vi "MeasLeakRate08.vi"() -> ()   [LabVIEW 2011]
panel:
  out "XY Graph":cluster{"Value":dbl[], "Value":dbl[]}(graph)
  in  "Control Valve local":bool
  in  "Exhaust Local":bool
  in  "Exhaust Close":bool
  in  "Exhaust Open":bool
  in  "Control Close":bool
  in  "Control Open":bool
  in  "reset":bool
  in  "# points to watch":i32=60
  out "leak rate (Torr/min)":string
  out "S20":dbl
  out "S11":dbl
  out "S10":dbl
  out "S01":dbl
  out "S00":dbl
  out "A11":dbl[](array[numeric])
  out "P":dbl
  in  "first":bool=TRUE
  out "A20":dbl[](array[numeric])
  out "A10":dbl[](array[numeric])
  out "A01":dbl[](array[numeric])
  out "A00":dbl[](array[numeric])
  in  "interval (s)":dbl=0.5
  in  "stop":bool
  out "P(Torr)":string
  # "Pressure control valve:"
  # "Exahaust valve:"
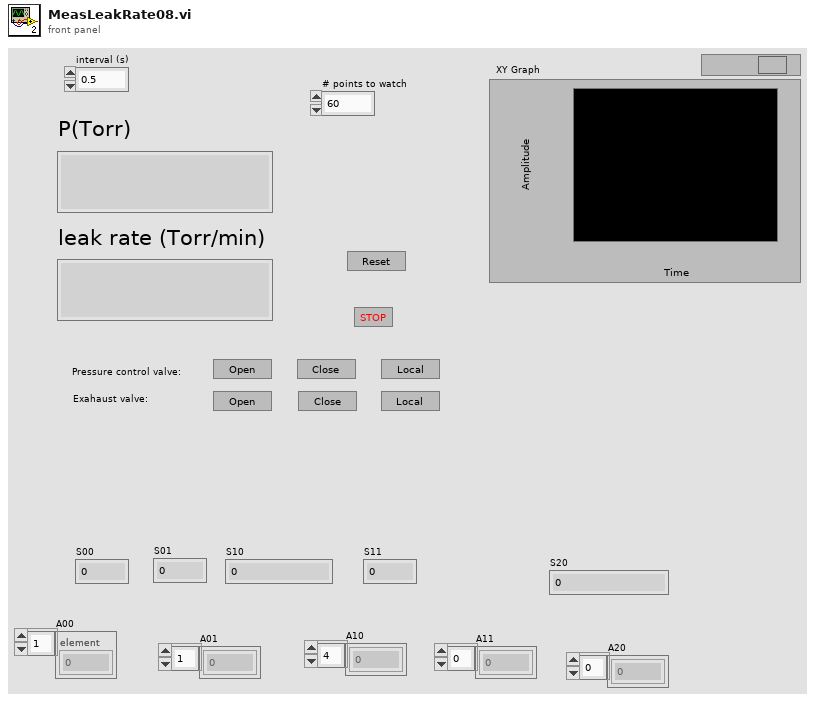
[diagram p1: front panel]
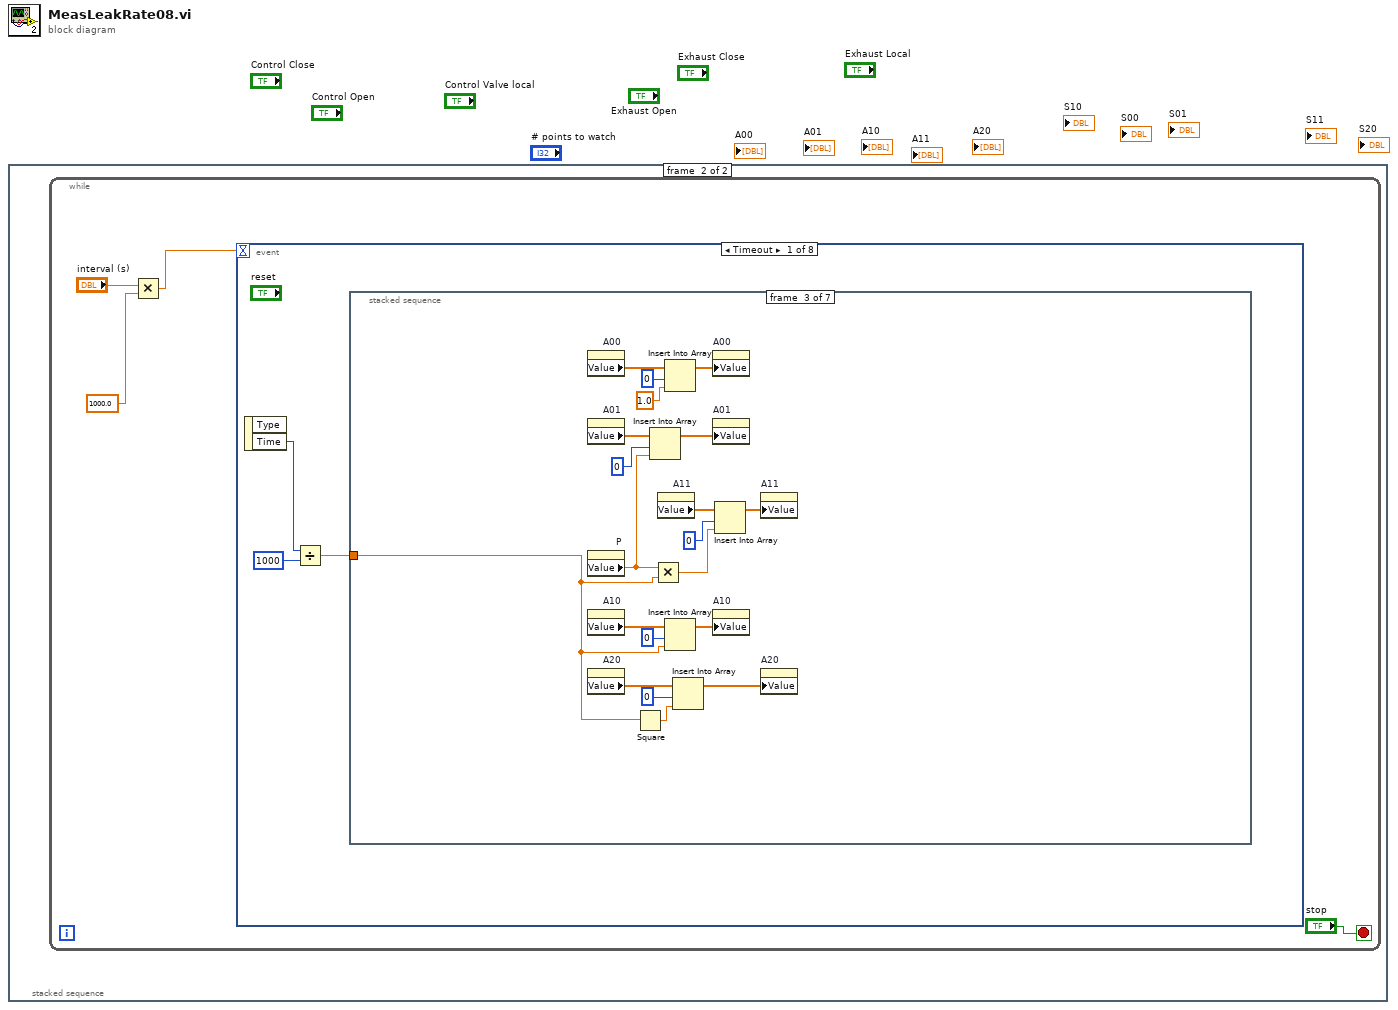
[diagram p0: block diagram]
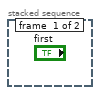
[diagram p2: hidden frame]
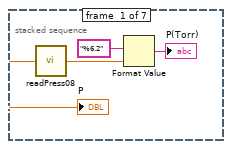
[diagram p3: hidden frame]
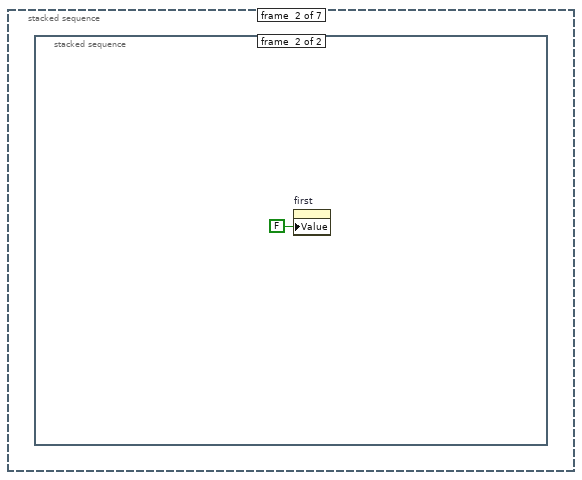
[diagram p4: hidden frame]
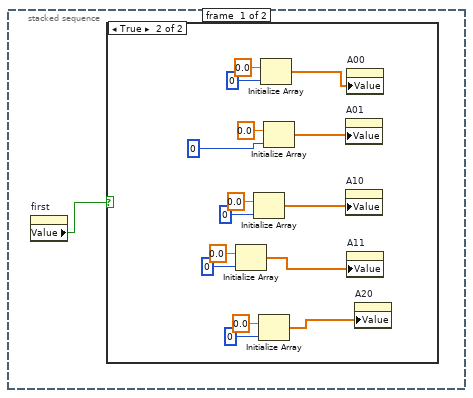
[diagram p5: hidden frame]
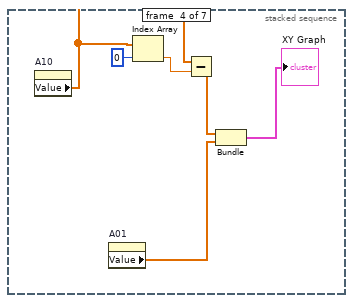
[diagram p7: hidden frame]
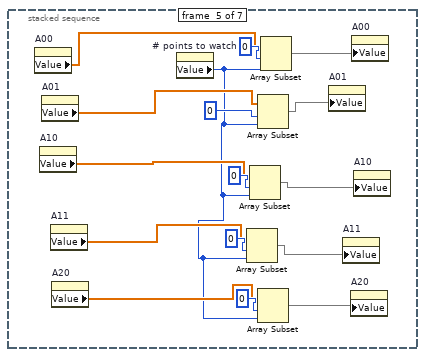
[diagram p8: hidden frame]
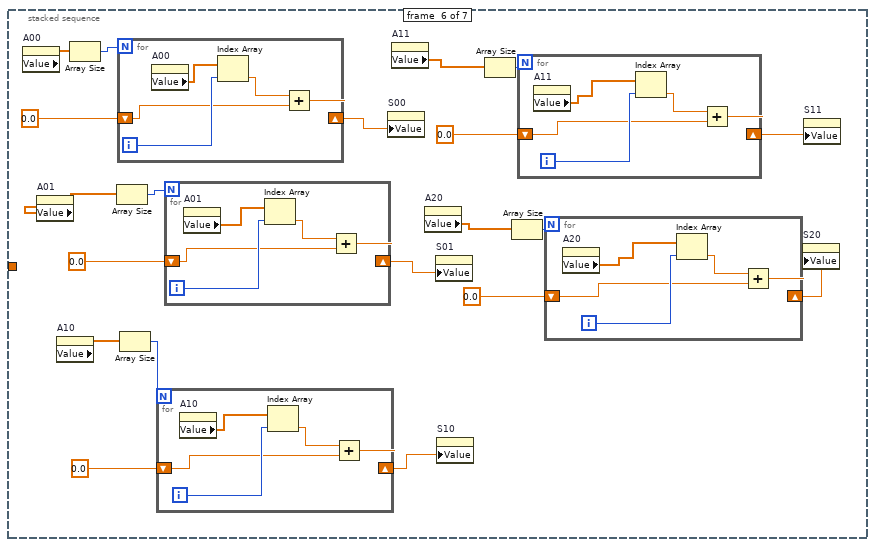
[diagram p9: hidden frame]
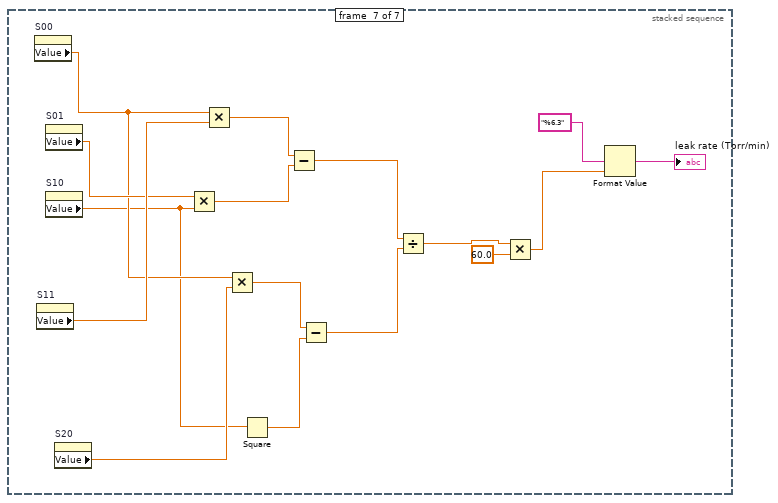
[diagram p10: hidden frame]
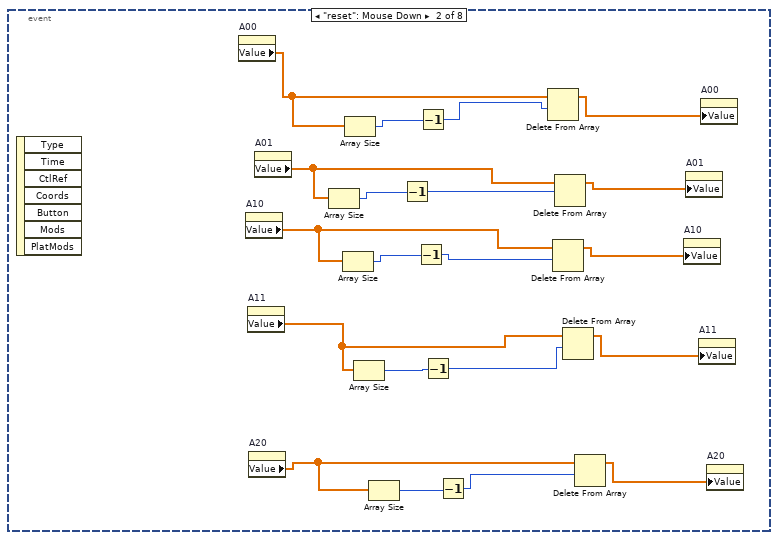
[diagram p11: hidden frame]
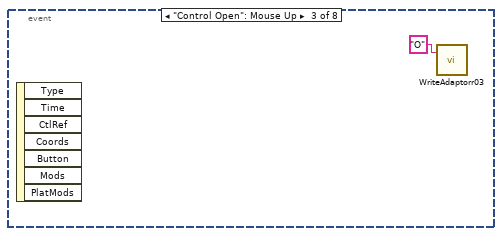
[diagram p12: hidden frame]
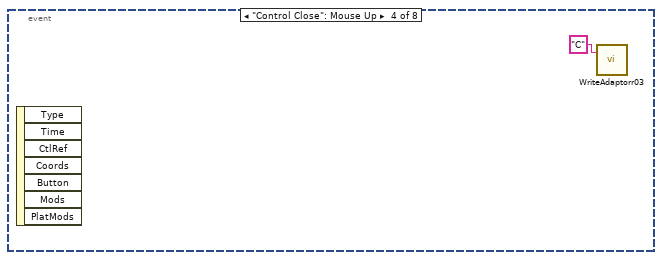
[diagram p13: hidden frame]
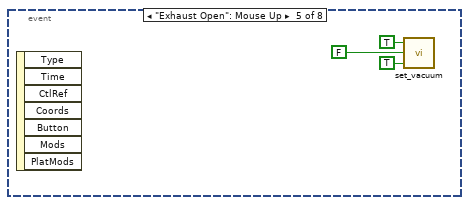
[diagram p14: hidden frame]
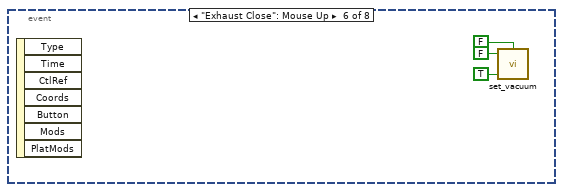
[diagram p15: hidden frame]
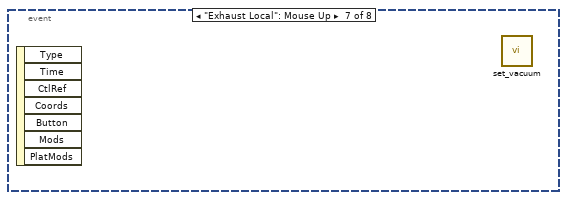
[diagram p16: hidden frame]
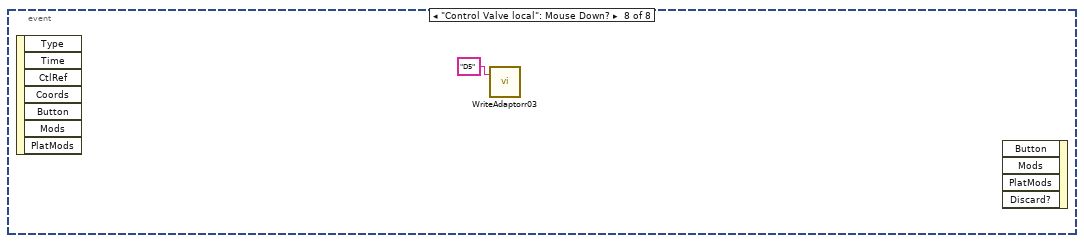
[diagram p17: hidden frame]
diagram:
  n1 = stacked-sequence {
    frame #0 {
    }
    frame #1 {
      n2 = while {
        stop <- "stop" stop-if-true
        n3 = Multiply(x="interval (s)", y=1000.0) -> (x*y=w2:dbl)
        n4 = event shown="[0] Timeout" {
          selector: _ -> [_ _ _ _ _ _ _ _]
          dyn-events: _ -> [_ _ _ _ _ _ _ _]
          timeout: w2 -> [_ _ _ _ _ _ _ _]
          event Timeout {
            n5 = event-data() -> ("Time"=w7:u32)  [unwired: 1 in, 1 out]
            n6 = Divide(x=w7, y=u32 1000) -> (x/y=w5:dbl)
            n7 = stacked-sequence {
              tunnel: w5 -> [_ _ w37 _ _ _ _]
              frame #0 {
                n8 = call "readPress08.vi"() -> ("P"=w9:dbl)
                "P" <- w9
                n9 = Format Value(format string="%6.2", value (0)=w9) -> (output string=→"P(Torr)":string)  [unwired: 1 in]
              }
              frame #1 {
                n10 = stacked-sequence {
                  frame #0 {
                    n11 = property on="first" class="Bool (strict)"() -> ("Value"=w11:bool)  [unwired: 2 in, 2 out]
                    n12 = case shown="True" w11 {
                      frame False {
                      }
                      frame True {
                        n13 = Initialize Array(0.0 ("element"), 0 ("dimension size")) -> (w14:dbl[])
                        n14 = Initialize Array(0.0 ("element"), 0 ("dimension size")) -> (w15:dbl[])
                        n15 = Initialize Array(0.0 ("element"), 0 ("dimension size")) -> (w13:dbl[])
                        n16 = Initialize Array(0.0 ("element"), 0 ("dimension size")) -> (w12:dbl[])
                        n17 = Initialize Array(0.0 ("element"), 0 ("dimension size")) -> (w16:dbl[])
                        n18 = property on="A01" class="Arr (strict)"("Value"=w16) -> ()  [unwired: 2 in, 2 out]
                        n19 = property on="A10" class="Arr (strict)"("Value"=w15) -> ()  [unwired: 2 in, 2 out]
                        n20 = property on="A00" class="Arr (strict)"("Value"=w12) -> ()  [unwired: 2 in, 2 out]
                        n21 = property on="A11" class="Arr (strict)"("Value"=w14) -> ()  [unwired: 2 in, 2 out]
                        n22 = property on="A20" class="Arr (strict)"("Value"=w13) -> ()  [unwired: 2 in, 2 out]
                      }
                    }
                  }
                  frame #1 {
                    n23 = property on="first" class="Bool (strict)"("Value"=FALSE ("first")) -> ()  [unwired: 2 in, 2 out]
                  }
                }
              }
              frame #2 {
                n24 = property on="A00" class="Arr (strict)"() -> ("Value"=w45:dbl[])  [unwired: 2 in, 2 out]
                n25 = property on="A01" class="Arr (strict)"() -> ("Value"=w43:dbl[])  [unwired: 2 in, 2 out]
                n26 = property on="P" class="DigNum (strict)"() -> ("Value"=w36:dbl)  [unwired: 2 in, 2 out]
                n27 = property on="A10" class="Arr (strict)"() -> ("Value"=w42:dbl[])  [unwired: 2 in, 2 out]
                n28 = property on="A20" class="Arr (strict)"() -> ("Value"=w40:dbl[])  [unwired: 2 in, 2 out]
                n29 = Square(x=w37) -> (x^2=w38:dbl)
                n30 = Insert Into Array(array=w43, index=0, new element=w36) -> (w28:dbl[])
                n31 = Multiply(x=w36, y=w37) -> (x*y=w34:dbl)
                n32 = property on="A11" class="Arr (strict)"() -> ("Value"=w35:dbl[])  [unwired: 2 in, 2 out]
                n33 = Insert Into Array(array=w45, index=0, new element=1.0 ("new element/subarray")) -> (w32:dbl[])
                n34 = Insert Into Array(array=w42, index=0, new element=w37) -> (w30:dbl[])
                n35 = Insert Into Array(array=w40, index=0, new element=w38) -> (w31:dbl[])
                n36 = property on="A00" class="Arr (strict)"("Value"=w32) -> ()  [unwired: 2 in, 2 out]
                n37 = property on="A01" class="Arr (strict)"("Value"=w28) -> ()  [unwired: 2 in, 2 out]
                n38 = property on="A10" class="Arr (strict)"("Value"=w30) -> ()  [unwired: 2 in, 2 out]
                n39 = Insert Into Array(array=w35, index=0, new element=w34) -> (w29:dbl[])
                n40 = property on="A11" class="Arr (strict)"("Value"=w29) -> ()  [unwired: 2 in, 2 out]
                n41 = property on="A20" class="Arr (strict)"("Value"=w31) -> ()  [unwired: 2 in, 2 out]
              }
              frame #3 {
                n42 = property on="A10" class="Arr (strict)"() -> ("Value"=w49:dbl[])  [unwired: 2 in, 2 out]
                n43 = property on="A01" class="Arr (strict)"() -> ("Value"=w52:dbl[])  [unwired: 2 in, 2 out]
                n44 = Index Array(array=w49, index=0) -> (element=w50:dbl)
                n45 = Subtract(x=w49, y=w50) -> (x-y=w48:dbl[])
                n46 = Bundle(w48, "Value"=w52) -> (→"XY Graph":cluster{dbl[], "Value":dbl[]})  [unwired: 1 in]
              }
              frame #4 {
                n47 = property on="A00" class="Arr (strict)"() -> ("Value"=w66:dbl[])  [unwired: 2 in, 2 out]
                n48 = property on="A10" class="Arr (strict)"() -> ("Value"=w60:dbl[])  [unwired: 2 in, 2 out]
                n49 = property on="A01" class="Arr (strict)"() -> ("Value"=w61:dbl[])  [unwired: 2 in, 2 out]
                n50 = property on="A11" class="Arr (strict)"() -> ("Value"=w59:dbl[])  [unwired: 2 in, 2 out]
                n51 = property on="A20" class="Arr (strict)"() -> ("Value"=w68:dbl[])  [unwired: 2 in, 2 out]
                n52 = property on="# points to watch" class="DigNum (strict)"() -> ("Value"=w54:i32)  [unwired: 2 in, 2 out]
                n53 = Array Subset(array=w59, index=0, length=w54) -> (w56:dbl[])
                n54 = Array Subset(array=w60, index=0, length=w54) -> (w57:dbl[])
                n55 = Array Subset(array=w61, index=0, length=w54) -> (w58:dbl[])
                n56 = Array Subset(array=w68, index=0, length=w54) -> (w55:dbl[])
                n57 = Array Subset(array=w66, index=0, length=w54) -> (w65:dbl[])
                n58 = property on="A01" class="Arr (strict)"("Value"=w58) -> ()  [unwired: 2 in, 2 out]
                n59 = property on="A11" class="Arr (strict)"("Value"=w56) -> ()  [unwired: 2 in, 2 out]
                n60 = property on="A20" class="Arr (strict)"("Value"=w55) -> ()  [unwired: 2 in, 2 out]
                n61 = property on="A00" class="Arr (strict)"("Value"=w65) -> ()  [unwired: 2 in, 2 out]
                n62 = property on="A10" class="Arr (strict)"("Value"=w57) -> ()  [unwired: 2 in, 2 out]
              }
              frame #5 {
                n63 = property on="A00" class="Arr (strict)"() -> ("Value"=w88:dbl[])  [unwired: 2 in, 2 out]
                n64 = property on="A01" class="Arr (strict)"() -> ("Value"=w84:dbl[])  [unwired: 2 in, 2 out]
                n65 = property on="A10" class="Arr (strict)"() -> ("Value"=w81:dbl[])  [unwired: 2 in, 2 out]
                n66 = Array Size(array=w88) -> (size(s)=w89:i32)
                n67 = Array Size(array=w84) -> (size(s)=w86:i32)
                n68 = for {
                  N: w89 -> [_]
                  shift-right: [w110] -> w74
                  shift-left: 0.0 -> [w111]
                  i -> [w113]
                  n69 = property on="A00" class="Arr (strict)"() -> ("Value"=w114:dbl[])  [unwired: 2 in, 2 out]
                  n70 = Index Array(array=w114, index=w113) -> (element=w112:dbl)
                  n71 = Add(x=w112, y=w111) -> (x+y=w110:dbl)
                }
                n72 = Array Size(array=w81) -> (size(s)=w83:i32)
                n73 = for {
                  N: w83 -> [_]
                  shift-right: [w101] -> w73
                  shift-left: 0.0 -> [w102]
                  i -> [w104]
                  n74 = property on="A10" class="Arr (strict)"() -> ("Value"=w100:dbl[])  [unwired: 2 in, 2 out]
                  n75 = Index Array(array=w100, index=w104) -> (element=w103:dbl)
                  n76 = Add(x=w103, y=w102) -> (x+y=w101:dbl)
                }
                n77 = for {
                  N: w86 -> [_]
                  shift-right: [w106] -> w72
                  shift-left: 0.0 -> [w107]
                  i -> [w109]
                  n78 = property on="A01" class="Arr (strict)"() -> ("Value"=w105:dbl[])  [unwired: 2 in, 2 out]
                  n79 = Index Array(array=w105, index=w109) -> (element=w108:dbl)
                  n80 = Add(x=w108, y=w107) -> (x+y=w106:dbl)
                }
                n81 = property on="S00" class="DigNum (strict)"("Value"=w74) -> ()  [unwired: 2 in, 2 out]
                n82 = property on="A11" class="Arr (strict)"() -> ("Value"=w78:dbl[])  [unwired: 2 in, 2 out]
                n83 = property on="A20" class="Arr (strict)"() -> ("Value"=w75:dbl[])  [unwired: 2 in, 2 out]
                n84 = property on="S01" class="DigNum (strict)"("Value"=w72) -> ()  [unwired: 2 in, 2 out]
                n85 = property on="S10" class="DigNum (strict)"("Value"=w73) -> ()  [unwired: 2 in, 2 out]
                n86 = Array Size(array=w78) -> (size(s)=w80:i32)
                n87 = Array Size(array=w75) -> (size(s)=w77:i32)
                n88 = for {
                  N: w80 -> [_]
                  shift-right: [w96] -> w71
                  shift-left: 0.0 -> [w97]
                  i -> [w99]
                  n89 = property on="A11" class="Arr (strict)"() -> ("Value"=w95:dbl[])  [unwired: 2 in, 2 out]
                  n90 = Index Array(array=w95, index=w99) -> (element=w98:dbl)
                  n91 = Add(x=w98, y=w97) -> (x+y=w96:dbl)
                }
                n92 = for {
                  N: w77 -> [_]
                  shift-right: [w91] -> w70
                  shift-left: 0.0 -> [w92]
                  i -> [w94]
                  n93 = property on="A20" class="Arr (strict)"() -> ("Value"=w90:dbl[])  [unwired: 2 in, 2 out]
                  n94 = Index Array(array=w90, index=w94) -> (element=w93:dbl)
                  n95 = Add(x=w93, y=w92) -> (x+y=w91:dbl)
                }
                n96 = property on="S20" class="DigNum (strict)"("Value"=w70) -> ()  [unwired: 2 in, 2 out]
                n97 = property on="S11" class="DigNum (strict)"("Value"=w71) -> ()  [unwired: 2 in, 2 out]
              }
              frame #6 {
                n98 = property on="S00" class="DigNum (strict)"() -> ("Value"=w126:dbl)  [unwired: 2 in, 2 out]
                n99 = property on="S11" class="DigNum (strict)"() -> ("Value"=w130:dbl)  [unwired: 2 in, 2 out]
                n100 = property on="S01" class="DigNum (strict)"() -> ("Value"=w129:dbl)  [unwired: 2 in, 2 out]
                n101 = property on="S10" class="DigNum (strict)"() -> ("Value"=w124:dbl)  [unwired: 2 in, 2 out]
                n102 = property on="S20" class="DigNum (strict)"() -> ("Value"=w125:dbl)  [unwired: 2 in, 2 out]
                n103 = Multiply(x=w129, y=w124) -> (x*y=w127:dbl)
                n104 = Multiply(x=w126, y=w130) -> (x*y=w128:dbl)
                n105 = Multiply(x=w126, y=w125) -> (x*y=w123:dbl)
                n106 = Square(x=w124) -> (x^2=w122:dbl)
                n107 = Subtract(x=w128, y=w127) -> (x-y=w121:dbl)
                n108 = Subtract(x=w123, y=w122) -> (x-y=w120:dbl)
                n109 = Divide(x=w121, y=w120) -> (x/y=w119:dbl)
                n110 = Multiply(x=w119, y=60.0) -> (x*y=w115:dbl)
                n111 = Format Value(format string="%6.3", value (0)=w115) -> (output string=→"leak rate (Torr/min)":string)  [unwired: 1 in]
              }
            }
          }
          event "reset": Mouse Down {
            n112 = event-data() -> ()  [unwired: 1 in, 7 out]
            n113 = property on="A00" class="Arr (strict)"() -> ("Value"=w150:dbl[])  [unwired: 2 in, 2 out]
            n114 = property on="A10" class="Arr (strict)"() -> ("Value"=w143:dbl[])  [unwired: 2 in, 2 out]
            n115 = property on="A11" class="Arr (strict)"() -> ("Value"=w140:dbl[])  [unwired: 2 in, 2 out]
            n116 = property on="A20" class="Arr (strict)"() -> ("Value"=w137:dbl[])  [unwired: 2 in, 2 out]
            n117 = property on="A01" class="Arr (strict)"() -> ("Value"=w146:dbl[])  [unwired: 2 in, 2 out]
            n118 = Array Size(array=w146) -> (size(s)=w145:i32)
            n119 = Array Size(array=w143) -> (size(s)=w142:i32)
            n120 = Array Size(array=w150) -> (size(s)=w148:i32)
            n121 = Array Size(array=w140) -> (size(s)=w139:i32)
            n122 = Array Size(array=w137) -> (size(s)=w136:i32)
            n123 = Decrement(x=w145) -> (x-1=w144:i32)
            n124 = Decrement(x=w142) -> (x-1=w141:i32)
            n125 = Decrement(x=w148) -> (x-1=w147:i32)
            n126 = Decrement(x=w139) -> (x-1=w138:i32)
            n127 = Decrement(x=w136) -> (x-1=w135:i32)
            n128 = Delete From Array(array=w150, length=w147) -> (array with subset deleted=w149:dbl[])  [unwired: 1 in, 1 out]
            n129 = Delete From Array(array=w143, length=w141) -> (array with subset deleted=w133:dbl[])  [unwired: 1 in, 1 out]
            n130 = Delete From Array(array=w146, length=w144) -> (array with subset deleted=w134:dbl[])  [unwired: 1 in, 1 out]
            n131 = Delete From Array(array=w140, length=w138) -> (array with subset deleted=w132:dbl[])  [unwired: 1 in, 1 out]
            n132 = Delete From Array(array=w137, length=w135) -> (array with subset deleted=w131:dbl[])  [unwired: 1 in, 1 out]
            n133 = property on="A10" class="Arr (strict)"("Value"=w133) -> ()  [unwired: 2 in, 2 out]
            n134 = property on="A01" class="Arr (strict)"("Value"=w134) -> ()  [unwired: 2 in, 2 out]
            n135 = property on="A11" class="Arr (strict)"("Value"=w132) -> ()  [unwired: 2 in, 2 out]
            n136 = property on="A00" class="Arr (strict)"("Value"=w149) -> ()  [unwired: 2 in, 2 out]
            n137 = property on="A20" class="Arr (strict)"("Value"=w131) -> ()  [unwired: 2 in, 2 out]
          }
          event "Control Open": Mouse Up {
            n138 = event-data() -> ()  [unwired: 1 in, 7 out]
            n139 = call "WriteAdaptorr03.vi"("string to write"="O") -> ()  [unwired: 1 in, 1 out]
          }
          event "Control Close": Mouse Up {
            n140 = event-data() -> ()  [unwired: 1 in, 7 out]
            n141 = call "WriteAdaptorr03.vi"("string to write"="C") -> ()  [unwired: 1 in, 1 out]
          }
          event "Exhaust Open": Mouse Up {
            n142 = event-data() -> ()  [unwired: 1 in, 7 out]
            n143 = call "set_vacuum.vi"("Vac Remote"=TRUE, "Atm Exhaust"=FALSE, "Vac Exhaust"=TRUE) -> ()
          }
          event "Exhaust Close": Mouse Up {
            n144 = event-data() -> ()  [unwired: 1 in, 7 out]
            n145 = call "set_vacuum.vi"("Vac Remote"=TRUE, "Atm Exhaust"=FALSE, "Vac Exhaust"=FALSE) -> ()
          }
          event "Exhaust Local": Mouse Up {
            n146 = event-data() -> ()  [unwired: 1 in, 7 out]
            n147 = call "set_vacuum.vi"() -> ()  [unwired: 3 in]
          }
          event "Control Valve local": Mouse Down? {
            n148 = event-data() -> ()  [unwired: 1 in, 7 out]
            n149 = call "WriteAdaptorr03.vi"("string to write"="D5") -> ()  [unwired: 1 in, 1 out]
            n150 = event-data() -> ()  [unwired: 5 in, 1 out]
          }
        }
      }
    }
  }
